vi "nrz二维转一维.vi"(1 "输入2维":dbl[][](array[numeric])) -> (0 "输出一维":dbl[](array[numeric]))   [LabVIEW 2013]
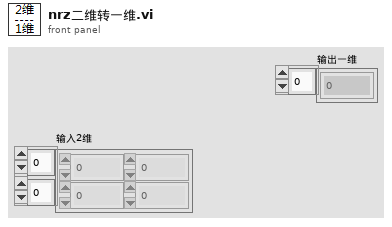
[diagram p1: front panel]
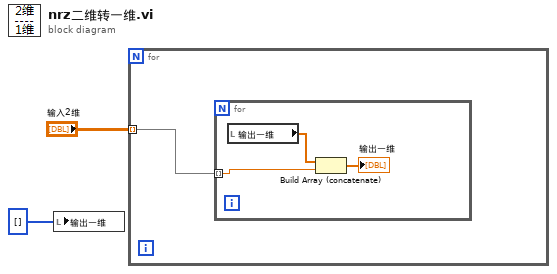
[diagram p0: block diagram]
diagram:
  n1 = local write "输出一维"(i32[] []) -> ()
  n2 = for {
    tunnel: "输入2维" -> [w3] mode=indexing
    n3 = for {
      tunnel: w3 -> [w6] mode=indexing
      n4 = local read "输出一维"() -> (w4:dbl[])
      n5 = Build Array (concatenate)(w4, w6) -> (→"输出一维":dbl[])
    }
  }
